vi "demo.vi"() -> ()   [LabVIEW 2021]
uses:
  DoublyLinkedList/DoublyLinkedList.lvclass
  Iterator/Iterator.lvclass
panel:
  out "data 3":dbl[](array[numeric])
  out "data 2":dbl[](array[numeric])
  out "error out":errorcluster
  out "data":dbl[](array[numeric])
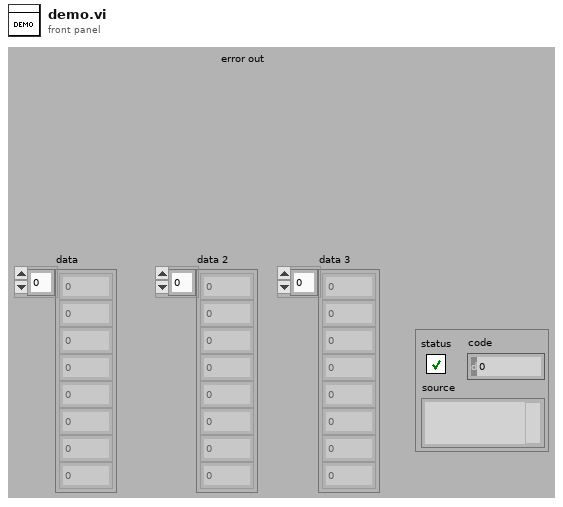
[diagram p1: front panel]
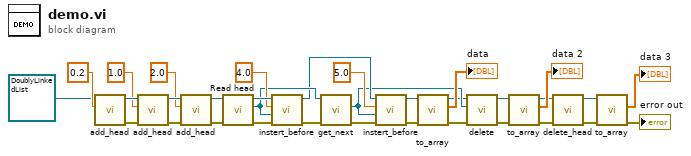
[diagram p0: block diagram]
diagram:
  n1 = call-dynamic "add_head.vi"("data"=0.2, "DoublyLinkedList in"=refnum<class "DoublyLinkedList.lvclass"> refnum ("DoublyLinkedList.lvclass")) -> ("error out"=w29:errorcluster, "DoublyLinkedList out"=w33:refnum<class "DoublyLinkedList.lvclass">)  [unwired: 8 in]
  n2 = call-dynamic "add_head.vi"("error in (no error)"=w29, "data"=1.0, "DoublyLinkedList in"=w33) -> ("error out"=w30:errorcluster, "DoublyLinkedList out"=w32:refnum<class "DoublyLinkedList.lvclass">)  [unwired: 7 in]
  n3 = call-dynamic "add_head.vi"("error in (no error)"=w30, "data"=2.0, "DoublyLinkedList in"=w32) -> ("error out"=w18:errorcluster, "DoublyLinkedList out"=w25:refnum<class "DoublyLinkedList.lvclass">)  [unwired: 7 in]
  n4 = call-dynamic "Read head.vi"("error in (no error)"=w18, "DoublyLinkedList in"=w25) -> ("error out"=w17:errorcluster, "DoublyNodeRef.lvclass"=w22:refnum<class "Iterator.lvclass">, "DoublyLinkedList out"=w24:refnum<class "DoublyLinkedList.lvclass">)  [unwired: 7 in]
  n5 = call-dynamic "instert_before.vi"("error in (no error)"=w17, "current node"=w22, "data"=4.0, "DoublyLinkedList in"=w24) -> ("error out"=w16:errorcluster, "DoublyLinkedList out"=w20:refnum<class "DoublyLinkedList.lvclass">)  [unwired: 6 in]
  n6 = call-dynamic "get_next.vi"("error in (no error)"=w16, "Iterator in"=w22) -> ("error out"=w15:errorcluster, "next"=w13:refnum<class "Iterator.lvclass">)  [unwired: 6 in, 2 out]
  n7 = call-dynamic "instert_before.vi"("error in (no error)"=w15, "current node"=w13, "data"=5.0, "DoublyLinkedList in"=w20) -> ("error out"=w14:errorcluster, "DoublyLinkedList out"=w19:refnum<class "DoublyLinkedList.lvclass">)  [unwired: 6 in]
  n8 = call-dynamic "to_array.vi"("error in (no error)"=w14, "List in"=w19) -> ("error out"=w11:errorcluster, "data"=→"data":dbl[], "List out"=w12:refnum<class "DoublyLinkedList.lvclass">)  [unwired: 7 in]
  n9 = call-dynamic "delete.vi"("error in (no error)"=w11, "current node"=w13, "DoublyLinkedList in"=w12) -> ("error out"=w10:errorcluster, "DoublyLinkedList out"=w9:refnum<class "DoublyLinkedList.lvclass">)  [unwired: 7 in]
  n10 = call-dynamic "to_array.vi"("error in (no error)"=w10, "List in"=w9) -> ("error out"=w6:errorcluster, "data"=→"data 2":dbl[], "List out"=w7:refnum<class "DoublyLinkedList.lvclass">)  [unwired: 7 in]
  n11 = call-dynamic "delete_head.vi"("error in (no error)"=w6, "DoublyLinkedList in"=w7) -> ("error out"=w5:errorcluster, "DoublyLinkedList out"=w4:refnum<class "DoublyLinkedList.lvclass">)  [unwired: 8 in]
  n12 = call-dynamic "to_array.vi"("error in (no error)"=w5, "List in"=w4) -> ("error out"=→"error out":errorcluster, "data"=→"data 3":dbl[])  [unwired: 7 in, 1 out]
